vi "$CTL_PropCtlr.vi"(8 "Pump Manual Controls":T1={"Pump Speed"=enum."STOP", "FILL"=FALSE, "Drain"=FALSE, "Auto/!Man"=TRUE, "Sim Level"=FALSE}, 9 "Pump Params":T3={"Empty Inches"=1.7, "Full Inches"=8.5, "RNG_SLOW"=0.5, "RNG_CREEP"=0.007, "RNG_STOP "=0.002, "VISA resource name"="COM4", "SPD_SLOW"=30, "SPD_CREEP"=7, "SPD_FAST"=100, "Zero template"=path "C:/AllenProjects/PWC-OLS/$Calibrtation/CAL_Level_RnR_241105.xlsx", "zero  Settle sec"=0.0} {"RNG_STOP" format="%#_13g"; "RNG_CREEP" format="%#_13g"; "RNG_SLOW" format="%#_13g"}, 10 "Level PV":dbl, 11 "Level SP":dbl) -> (1 "Pump Speed Out":T2=enum."STOP", 2 "X< Neg":bool, 3 "X>Pos":bool, 5 "Neg <X<Pos":bool=TRUE)   [LabVIEW 2024]
uses:
  Control Definitions/Def_PumpSpeed.ctl
  Control Definitions/DEF_PumpParams.ctl
  Control Definitions/DEF_PumpManCtl.ctl
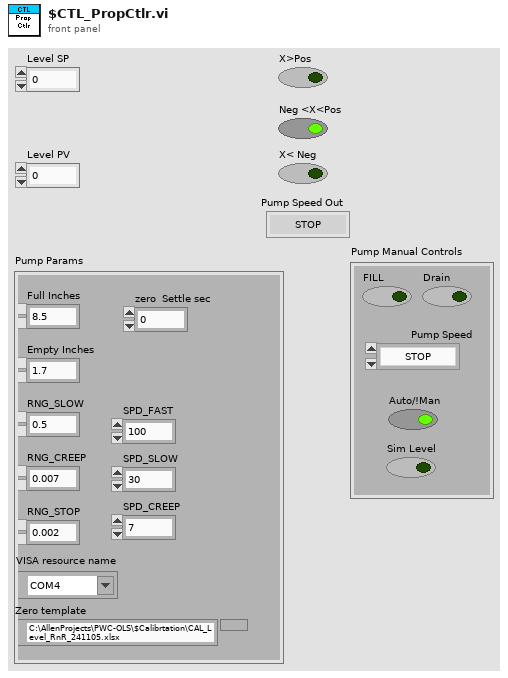
[diagram p1: front panel]
types:
  T1 = typedef "DEF_PumpManCtl.ctl" = cluster{"Pump Speed":T2, "FILL":bool, "Drain":bool, "Auto/!Man":bool, "Sim Level":bool}
  T2 = typedef "Def_PumpSpeed.ctl" = enum16{"FAST", "SLOW", "CREEP", "STOP"}
  T3 = typedef "DEF_PumpParams.ctl" = cluster{"Empty Inches":dbl, "Full Inches":dbl, "RNG_SLOW":dbl, "RNG_CREEP":dbl, "RNG_STOP ":dbl, "VISA resource name":refnum<visa-resource-name>, "SPD_SLOW":i32, "SPD_CREEP":i32, "SPD_FAST":i32, "Zero template":path, "zero  Settle sec":dbl}
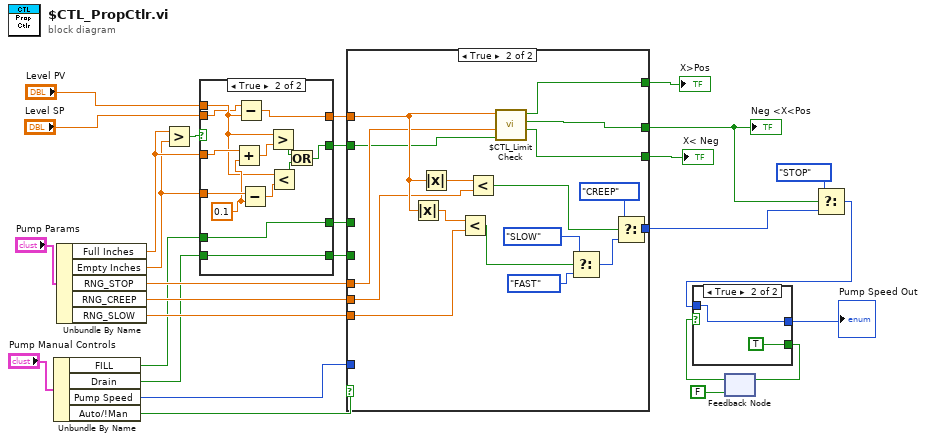
[diagram p0: block diagram]
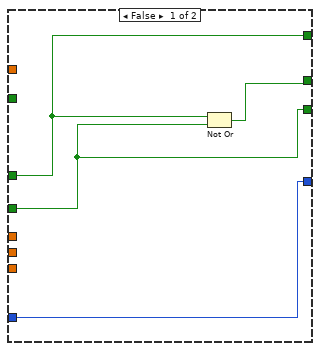
[diagram p2: hidden frame]
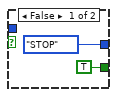
[diagram p3: hidden frame]
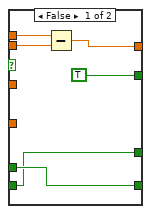
[diagram p4: hidden frame]
diagram:
  n1 = Unbundle By Name("Pump Manual Controls") -> ("FILL"=w4:bool, "Drain"=w2:bool, "Pump Speed"=w5:T2, "Auto/!Man"=w6:bool)
  n2 = Unbundle By Name("Pump Params") -> ("Full Inches"=w11:dbl, "Empty Inches"=w10:dbl, "RNG_STOP"=w12:dbl, "RNG_CREEP"=w13:dbl, "RNG_SLOW"=w14:dbl)
  n3 = Greater?(x=w11, y=w10) -> (0:w16:bool)
  n4 = case shown="True" w16 {
    tunnel: [w34 w47] -> w24
    tunnel: "Level PV" -> [w33 w36]
    tunnel: "Level SP" -> [w32 w35]
    tunnel: w11 -> [_ w40]
    tunnel: w10 -> [_ w43]
    tunnel: [TRUE w44] -> w8
    tunnel: w4 -> [w30 w38]
    tunnel: [w29 w38] -> w3
    tunnel: w2 -> [w29 w37]
    tunnel: [w30 w37] -> w1
    frame False {
      n5 = Subtract(x=w33, y=w32) -> (x-y=w34:dbl)
    }
    frame True {
      w39 = 0.1 ("y")
      n6 = Add(x=w40, y=w39) -> (x+y=w41:dbl)
      n7 = Subtract(x=w35, y=w36) -> (x-y=w47:dbl)
      n8 = Subtract(x=w43, y=w39) -> (x-y=w42:dbl)
      n9 = Greater?(x=w36, y=w41) -> (0:w45:bool)
      n10 = Less?(x=w36, y=w42) -> (x < y?=w46:bool)
      n11 = Or(x=w45, y=w46) -> (x .or. y?=w44:bool)
    }
  }
  n12 = case shown="True" w6 {
    tunnel: [w50 w66] -> w28
    tunnel: [w49 w65] -> w25
    tunnel: w24 -> [_ w61]
    tunnel: [w51 w57] -> w22
    tunnel: w14 -> [_ w56]
    tunnel: w13 -> [_ w55]
    tunnel: w12 -> [_ w54]
    tunnel: [w48 w53] -> w9
    tunnel: w8 -> [_ w52]
    tunnel: w5 -> [w51 _]
    tunnel: w3 -> [w50 _]
    tunnel: w1 -> [w49 _]
    frame False {
      n13 = Not Or(1:w49, 2:w50) -> (0:w48:bool)
    }
    frame True {
      n14 = Absolute Value(x=w61) -> (abs(x)=w67:dbl)
      n15 = Absolute Value(x=w61) -> (abs(x)=w62:dbl)
      n16 = Less?(x=w67, y=w56) -> (x < y?=w68:bool)
      n17 = Less?(x=w62, y=w55) -> (x < y?=w64:bool)
      n18 = call "$CTL_Limit Check.vi"("E-Stop"=w52, "Limit"=w54, "X"=w61) -> ("X< Neg"=w65:bool, "Neg <X<Pos"=w53:bool, "X>Pos"=w66:bool)  [unwired: 6 in]
      n19 = Select(t=Def_PumpSpeed."SLOW" ("Pump Speed"), s=w68, f=Def_PumpSpeed."FAST") -> (s? t:f=w59:T2)
      n20 = Select(t=Def_PumpSpeed."CREEP" ("Pump Speed"), s=w64, f=w59) -> (s? t:f=w57:T2)
    }
  }
  "X>Pos" <- w28
  "X< Neg" <- w25
  "Neg <X<Pos" <- w9
  n21 = feedback #1(FALSE) -> (w21:bool)
  n22 = Select(t=Def_PumpSpeed."STOP" ("Pump Speed"), s=w9, f=w22) -> (s? t:f=w17:T2)
  n23 = case shown="True" w21 {
    tunnel: [TRUE TRUE] -> w20
    tunnel: [Def_PumpSpeed."STOP" ("Pump Speed") w71] -> w18
    tunnel: w17 -> [_ w71]
    frame False {
    }
    frame True {
    }
  }
  "Pump Speed Out" <- w18
  n24 = feedback-in #1(w20) -> ()
